vi "Generate Poll List.vi"(7 "MaxPollGap":i32=16, 11 "IO List":cluster{"ModbusRef":u32, "ModbusDataType":T2}[](array[cluster])) -> (3 "Poll List":T1[](array[typedef]))   [LabVIEW 2018, in "MB PLC Client.lvlib"]
doc: "Generate the poll list based on a list of IO points (modbus starting ref and data type).\n\nUse Max Poll Gap to specify the maximum number registers to read between IO points. This is useful for reducing the number of Mobus transactions per polling cycle."
uses:
  MB PLC Client.lvlib
  Types/MB Data Types_Enum.ctl
  Types/MB Ref Range_Cluster.ctl
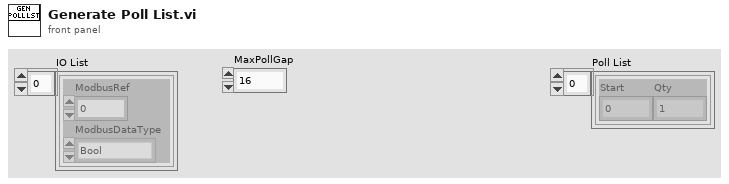
[diagram p1: front panel]
types:
  T1 = typedef "MB PLC Client.lvlib/MB Ref Range_Cluster.ctl" = cluster{"Start":u32, "Qty":u16}
  T2 = typedef "MB PLC Client.lvlib/MB Data Types_Enum.ctl" = enum16{"Bool", "U16", "U32", "I16", "I32", "SGL", "DBL"}
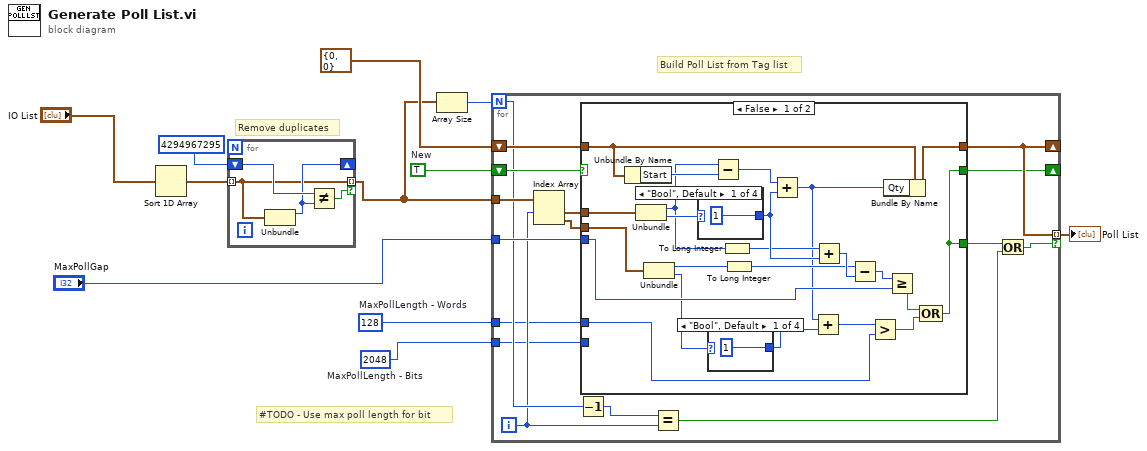
[diagram p0: block diagram]
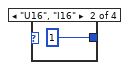
[diagram p2: hidden frame]
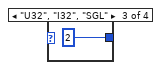
[diagram p3: hidden frame]
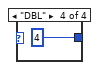
[diagram p4: hidden frame]
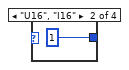
[diagram p5: hidden frame]
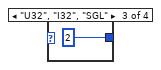
[diagram p6: hidden frame]
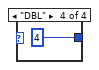
[diagram p7: hidden frame]
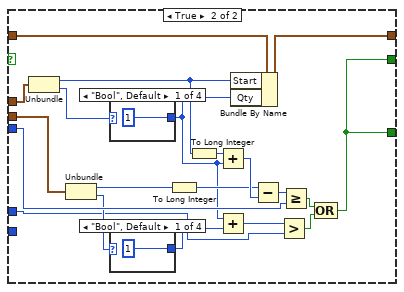
[diagram p8: hidden frame]
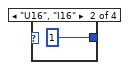
[diagram p9: hidden frame]
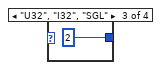
[diagram p10: hidden frame]
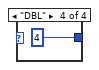
[diagram p11: hidden frame]
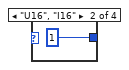
[diagram p12: hidden frame]
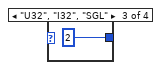
[diagram p13: hidden frame]
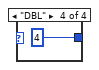
[diagram p14: hidden frame]
diagram:
  w2 = 2048  # MaxPollLength - Bits
  w3 = u16 128  # MaxPollLength - Words
  w9 = TRUE  # New
  # "#TODO - Use max poll length for bit"
  # "Build Poll List from Tag list"
  # "Remove duplicates"
  n1 = Sort 1D Array(array="IO List") -> (sorted array=w6:cluster{"ModbusRef":u32, "ModbusDataType":T2}[])
  n2 = for {
    tunnel: w6 -> [w13] mode=indexing
    shift-right: [w14] -> _
    shift-left: u32 4294967295 ("ModbusRef") -> [w15]
    tunnel: [w13] -> w4 mode=indexing if=w12
    n3 = Unbundle(w13) -> ("ModbusRef"=w14:u32)  [unwired: 1 out]
    n4 = Not Equal?(x=w15, y=w14) -> (x != y?=w12:bool)
  }
  n5 = Array Size(array=w4) -> (size(s)=w7:i32)
  n6 = for {
    N: w7 -> [w22]
    shift-right: [w25] -> _
    shift-left: T1 {"Start"=0, "Qty"=0} ("Cluster") -> [w30]
    tunnel: "MaxPollGap" -> [w29]
    tunnel: w4 -> [w28]
    shift-right: [w24] -> _
    shift-left: w9 -> [w31]
    tunnel: [w25] -> w1 mode=indexing if=w18
    tunnel: w3 -> [w17]
    tunnel: w2 -> [w16]
    i -> [w20]
    n7 = Index Array(array=w28, index #1=w20) -> (element #1=w27:cluster{"ModbusRef":u32, "ModbusDataType":T2}, element #2=w26:cluster{"ModbusRef":u32, "ModbusDataType":T2})  [unwired: 1 in]
    n8 = Decrement(x=w22) -> (x-1=w21:i32)
    n9 = case shown="False" w31 {
      tunnel: w27 -> [w54 w82]
      tunnel: w30 -> [w49 w81]
      tunnel: [w48 w79] -> w25
      tunnel: w29 -> [w42 w75]
      tunnel: w26 -> [w53 w78]
      tunnel: [w32 w63] -> w23
      tunnel: [w32 w63] -> w24
      tunnel: w17 -> [w35 w66]
      tunnel: w16 -> [_ _]
      frame False {
        n10 = Unbundle By Name(w49) -> ("Start"=w52:u32)
        n11 = Unbundle(w54) -> ("ModbusRef"=w47:u32, "ModbusDataType"=w51:T2)
        n12 = Unbundle(w53) -> ("ModbusRef"=w45:u32, "ModbusDataType"=w39:T2)
        n13 = case shown="\"Bool\", Default" w51 {
          tunnel: [u16 1 u16 1 u16 2 u16 4] -> w46
          frame "Bool", Default {
          }
          frame "U16", "I16" {
          }
          frame "U32", "I32", "SGL" {
          }
          frame "DBL" {
          }
        }
        n14 = case shown="\"Bool\", Default" w39 {
          tunnel: [u16 1 u16 1 u16 2 u16 4] -> w37
          frame "Bool", Default {
          }
          frame "U16", "I16" {
          }
          frame "U32", "I32", "SGL" {
          }
          frame "DBL" {
          }
        }
        n15 = Subtract(x=w47, y=w52) -> (x-y=w50:u32)
        n16 = To Long Integer(number=w47) -> (32bit integer=w40:i32)
        n17 = To Long Integer(number=w45) -> (32bit integer=w41:i32)
        n18 = Add(x=w50, y=w46) -> (x+y=w38:u32)
        n19 = Add(x=w38, y=w37) -> (x+y=w36:u32)
        n20 = Add(x=w40, y=w46) -> (x+y=w44:i32)
        n21 = Subtract(x=w41, y=w44) -> (x-y=w43:i32)
        n22 = Greater?(x=w36, y=w35) -> (0:w33:bool)
        n23 = Bundle By Name(cluster=w49, "Qty"=w38) -> (w48:T1)
        n24 = Greater Or Equal?(x=w43, y=w42) -> (x >= y?=w34:bool)
        n25 = Compound Arithmetic op=OR(w34, w33) -> (w32:bool)
      }
      frame True {
        n26 = Unbundle(w82) -> ("ModbusRef"=w72:u32, "ModbusDataType"=w80:T2)
        n27 = Unbundle(w78) -> ("ModbusRef"=w77:u32, "ModbusDataType"=w69:T2)
        n28 = case shown="\"Bool\", Default" w80 {
          tunnel: [u16 1 u16 1 u16 2 u16 4] -> w70
          frame "Bool", Default {
          }
          frame "U16", "I16" {
          }
          frame "U32", "I32", "SGL" {
          }
          frame "DBL" {
          }
        }
        n29 = case shown="\"Bool\", Default" w69 {
          tunnel: [u16 1 u16 1 u16 2 u16 4] -> w68
          frame "Bool", Default {
          }
          frame "U16", "I16" {
          }
          frame "U32", "I32", "SGL" {
          }
          frame "DBL" {
          }
        }
        n30 = To Long Integer(number=w77) -> (32bit integer=w73:i32)
        n31 = To Long Integer(number=w72) -> (32bit integer=w71:i32)
        n32 = Add(x=w71, y=w70) -> (x+y=w74:i32)
        n33 = Add(x=w70, y=w68) -> (x+y=w67:u16)
        n34 = Bundle By Name(cluster=w81, "Start"=w72, "Qty"=w70) -> (w79:T1)
        n35 = Subtract(x=w73, y=w74) -> (x-y=w76:i32)
        n36 = Greater?(x=w67, y=w66) -> (0:w64:bool)
        n37 = Greater Or Equal?(x=w76, y=w75) -> (x >= y?=w65:bool)
        n38 = Compound Arithmetic op=OR(w65, w64) -> (w63:bool)
      }
    }
    n39 = Equal?(x=w21, y=w20) -> (x = y?=w19:bool)
    n40 = Or(x=w23, y=w19) -> (x .or. y?=w18:bool)
  }
  "Poll List" <- w1
